vi "global get findinput.vi"() -> ()   [LabVIEW 2014]
panel:
  in  "KV result output y":dbl format="%.5p"
  in  "KV output 2 y":dbl format="%.5p"
  in  "KV output 1 y":dbl format="%.5p"
  in  "KV input 2 y":dbl format="%.5p"
  in  "KV input 1 y":dbl format="%.5p"
  in  "KV result output x":dbl format="%.5p"
  in  "KV output 2 x":dbl format="%.5p"
  in  "KV output 1 x":dbl format="%.5p"
  in  "KV input 2 x":dbl format="%.5p"
  in  "KV input 1 x":dbl format="%.5p"
  in  "W result output y":dbl format="%.5p"
  in  "W output 2 y":dbl format="%.5p"
  in  "W output 1 y":dbl format="%.5p"
  in  "W input 2 y":dbl format="%.5p"
  in  "W input 1 y":dbl format="%.5p"
  in  "W result output x":dbl format="%.5p"
  in  "W output 2 x":dbl format="%.5p"
  in  "W output 1 x":dbl format="%.5p"
  in  "W input 2 x":dbl format="%.5p"
  in  "W input 1 x":dbl format="%.5p"
  in  "1R result output y":dbl format="%.5p"
  in  "1R output 2 y":dbl format="%.5p"
  in  "1R output 1 y":dbl format="%.5p"
  in  "1R input 2 y":dbl format="%.5p"
  in  "1R input 1 y":dbl format="%.5p"
  in  "1R result output x":dbl format="%.5p"
  in  "1R output 2 x":dbl format="%.5p"
  in  "1R output 1 x":dbl format="%.5p"
  in  "1R input 2 x":dbl format="%.5p"
  in  "1R input 1 x":dbl format="%.5p"
  in  "10R result output y":dbl format="%.5p"
  in  "10R output 2 y":dbl format="%.5p"
  in  "10R output 1 y":dbl format="%.5p"
  in  "10R input 2 y":dbl format="%.5p"
  in  "10R input 1 y":dbl format="%.5p"
  in  "10R result output x":dbl format="%.5p"
  in  "10R output 2 x":dbl format="%.5p"
  in  "10R output 1 x":dbl format="%.5p"
  in  "10R input 2 x":dbl format="%.5p"
  in  "10R input 1 x":dbl format="%.5p"
  in  "AD result output y":dbl format="%.5p"
  in  "AD output 2 y":dbl format="%.5p"
  in  "AD output 1 y":dbl format="%.5p"
  in  "AD input 2 y":dbl format="%.5p"
  in  "AD input 1 y":dbl format="%.5p"
  in  "AD result output x":dbl format="%.5p"
  in  "AD output 2 x":dbl format="%.5p"
  in  "AD output 1 x":dbl format="%.5p"
  in  "AD input 2 x":dbl format="%.5p"
  in  "AD input 1 x":dbl format="%.5p"
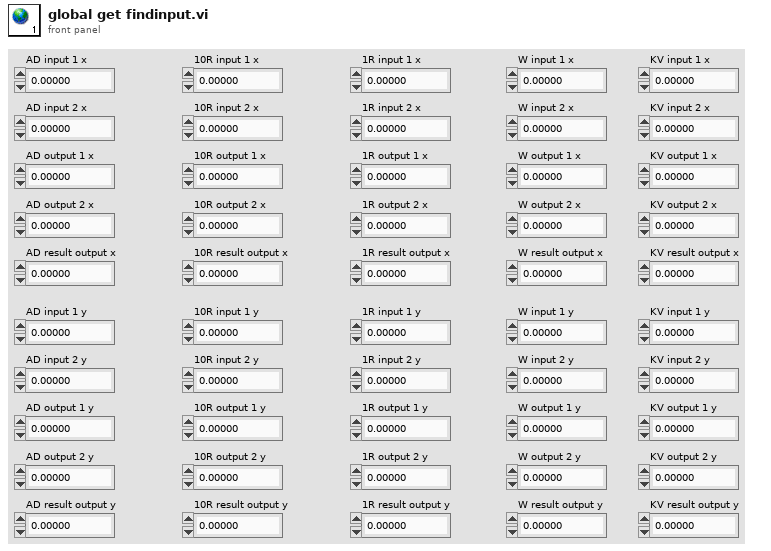
[diagram p1: front panel]
diagram:
